vi "Remove from Wire.vi"(8 "error in (no error)":errorcluster, 10 "Output Term":refnum<vi>, 11 "Input Term":refnum<vi>) -> (0 "error out":errorcluster)   [LabVIEW 2014]
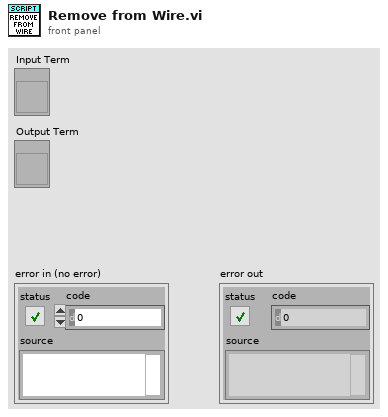
[diagram p1: front panel]
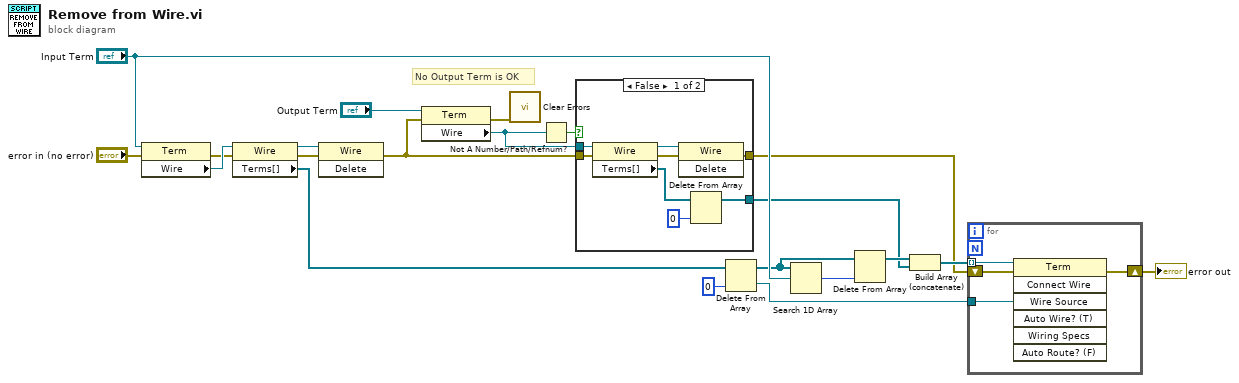
[diagram p0: block diagram]
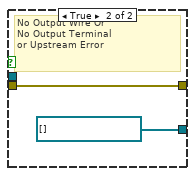
[diagram p2: hidden frame]
diagram:
  # "No Output Term is OK"
  n1 = property class="Term"(reference="Input Term", error in="error in (no error)") -> (error out=w18:errorcluster, "Wire"=w19:refnum<vi>)  [unwired: 1 out]
  n2 = property class="Wire"(reference=w19, error in=w18) -> (reference out=w10:refnum<vi>, error out=w6:errorcluster, "Terms[]"=w7:refnum<vi>[])
  n3 = invoke class="Wire" method="Delete"(reference=w10, error in=w6) -> (error out=w4:errorcluster)  [unwired: 1 in, 2 out]
  n4 = property class="Term"(reference="Output Term", error in=w4) -> (error out=w2:errorcluster, "Wire"=w5:refnum<vi>)  [unwired: 1 out]
  n5 = call <vilib>:"Clear Errors.vi"("error in (no error)"=w2) -> ()  [unwired: 5 in, 2 out]
  n6 = Not A Number/Path/Refnum?(number/path/refnum=w5) -> (NaN/Path/Refnum?=w3:bool)
  n7 = case shown="False" w3 {
    tunnel: w4 -> [w29 w31]
    tunnel: w5 -> [w28 _]
    tunnel: [w26 w31] -> w9
    tunnel: [w22 refnum<vi>[] [] ("Terms[]")] -> w1
    frame False {
      n8 = property class="Wire"(reference=w28, error in=w29) -> (reference out=w27:refnum<vi>, error out=w25:errorcluster, "Terms[]"=w23:refnum<vi>[])
      n9 = invoke class="Wire" method="Delete"(reference=w27, error in=w25) -> (error out=w26:errorcluster)  [unwired: 1 in, 2 out]
      n10 = Delete From Array(array=w23, index=0) -> (array with subset deleted=w22:refnum<vi>[])  [unwired: 1 in, 1 out]
    }
    frame True {
      # "No Output Wire Or\nNo Output Terminal\nor Upstream Error"
    }
  }
  n11 = Delete From Array(array=w7, index=0) -> (deleted portion=w11:refnum<vi>, array with subset deleted=w14:refnum<vi>[])  [unwired: 1 in]
  n12 = Search 1D Array(1D array=w14, element="Input Term") -> (index of element=w16:i32)  [unwired: 1 in]
  n13 = Delete From Array(array=w14, index=w16) -> (array with subset deleted=w12:refnum<vi>[])  [unwired: 1 in, 1 out]
  n14 = Build Array (concatenate)(w12, w1) -> (w13:refnum<vi>[])
  n15 = for {
    shift-right: [w35] -> w21
    shift-left: w9 -> [w34]
    tunnel: w13 -> [w33] mode=indexing
    tunnel: w11 -> [w32]
    n16 = invoke class="Term" method="Connect Wire"(reference=w33, error in=w34, "Wire Source"=w32) -> (error out=w35:errorcluster)  [unwired: 4 in, 6 out]
  }
  "error out" <- w21
